vi "Load Controller Type from Path.vi"(2 "error in (no error)":errorcluster, 3 "Absolute Path":path) -> (0 "error out":errorcluster, 1 "Controller out":refnum<class "Generic Plugin.lvclass">)   [LabVIEW 2020, in "Generic Plugin.lvclass"]
uses:
  Generic Plugin.lvclass
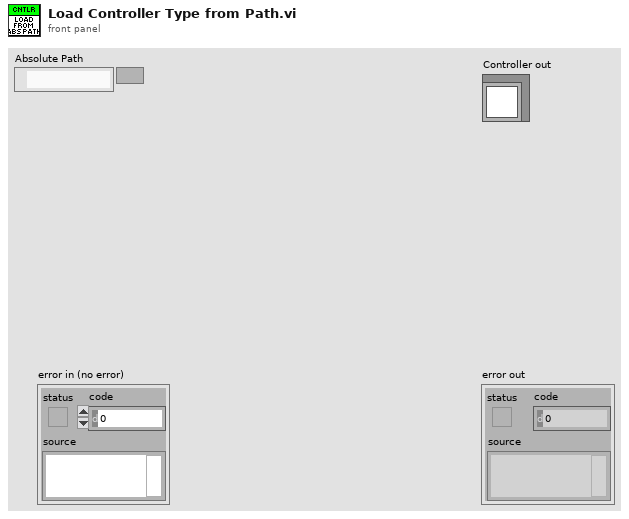
[diagram p1: front panel]
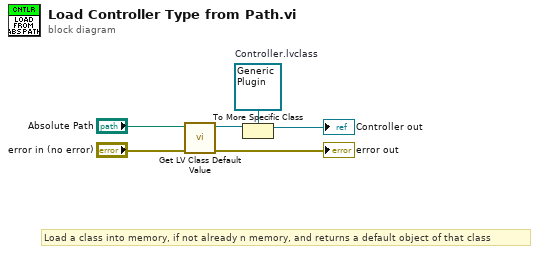
[diagram p0: block diagram]
diagram:
  w2 = refnum<class "Generic Plugin.lvclass"> refnum  # Controller.lvclass
  # "Load a class into memory, if not already n memory, and returns a default object of that class"
  n1 = call <vilib>:"Get LV Class Default Value.vi"("error in (no error)"="error in (no error)", "class path"="Absolute Path") -> ("error out"=→"error out":errorcluster, "object"=w3:refnum<class>)  [unwired: 8 in]
  n2 = To More Specific Class(target class=w2, reference=w3) -> (specific class reference=→"Controller out":refnum<class "Generic Plugin.lvclass">)  [unwired: 1 in, 1 out]
